vi "Get Station Config Settings.vi"(8 "error in (no error)":errorcluster, 11 "Station Config in":refnum<class "Station Config.lvclass">) -> (0 "error out":errorcluster, 3 "Station Settings":T1)   [LabVIEW 2017, in "Station Config.lvlib" / "Station Config.lvclass"]
uses:
  Station Config.lvclass
  Station Settings -- Cluster.ctl
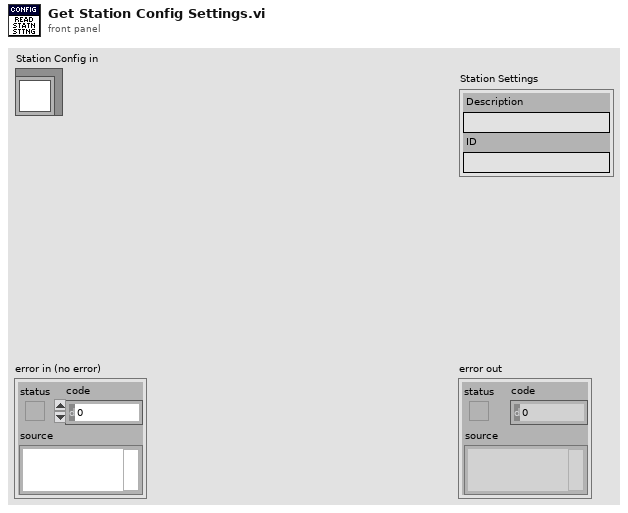
[diagram p1: front panel]
types:
  T1 = typedef "Station Config.lvlib/Station Config.lvclass/Station Settings -- Cluster.ctl" = cluster{"Description":string, "ID":string}
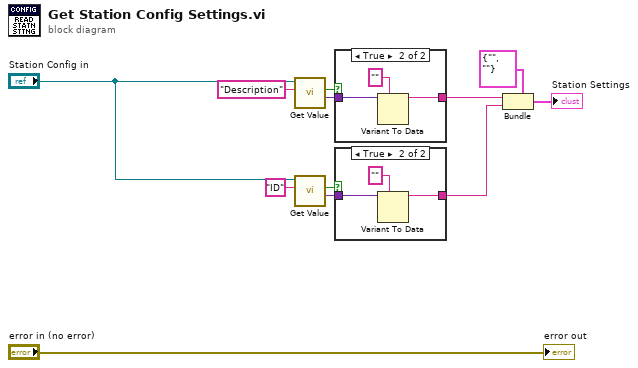
[diagram p0: block diagram]
diagram:
  n1 = call-dynamic "Get Value.vi"("Key"="Description", "Registry in"="Station Config in") -> ("Value"=w10:variant, "found?"=w11:bool)  [unwired: 6 in, 2 out]
  n2 = call-dynamic "Get Value.vi"("Key"="ID", "Registry in"="Station Config in") -> ("Value"=w7:variant, "found?"=w6:bool)  [unwired: 6 in, 2 out]
  n3 = case shown="True" w11 {
    tunnel: w10 -> [_ w15]
    tunnel: [_ w14] -> w4
    frame False {
    }
    frame True {
      n4 = Variant To Data(type="", Variant=w15) -> (data=w14:string)  [unwired: 1 in, 1 out]
    }
  }
  n5 = case shown="True" w6 {
    tunnel: w7 -> [_ w18]
    tunnel: [_ w17] -> w3
    frame False {
    }
    frame True {
      n6 = Variant To Data(type="", Variant=w18) -> (data=w17:string)  [unwired: 1 in, 1 out]
    }
  }
  n7 = Bundle(cluster=T1 {"Description"="", "ID"=""} ("Cluster"), "Description"=w4, "ID"=w3) -> (→"Station Settings":T1)
  "error out" <- "error in (no error)"
